vi "SYSKON P4500 Init Config.vi"() -> ()   [LabVIEW 2010]
panel:
  out "Output Current":string
  out "Output Voltage":string
  in  "Output State":bool=TRUE
  in  "Baud Rate":u32=19200
  in  "OCP Level":dbl=32.0 format="%.3f"
  in  "OVP Level":dbl=24.0 format="%.3f"
  in  "Instr. Descriptor":refnum<visa-resource-name>="COM4"
  out "error out":errorcluster {"code" format="%x"}
  in  "error in":errorcluster {"code" format="%x"}
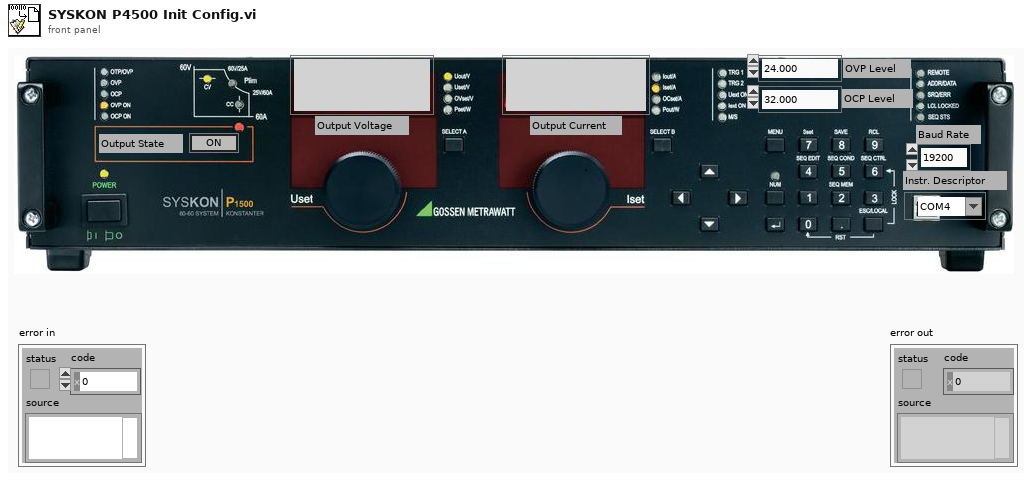
[diagram p1: front panel]
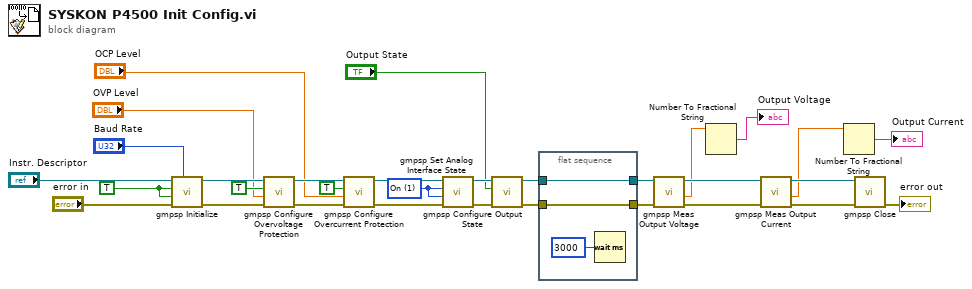
[diagram p0: block diagram]
diagram:
  w21 = 1 items=["Off", "On", "Signal State"] ("U ext (0: Off)")
  w31 = TRUE ("ID Query (True)")
  n1 = call <instrlib>:"gmpsp Initialize.vi"("Baud Rate"="Baud Rate", "error in"="error in", "Reset (True)"=w31, "ID Query (True)"=w31, "Instr. Descriptor"="Instr. Descriptor") -> ("error out"=w27:errorcluster, "VISA resource name out"=w29:refnum<visa-resource-name>)  [unwired: 5 in]
  n2 = call <instrlib>:"gmpsp Configure Overvoltage Protection.vi"("error in (no error)"=w27, "OVP Level (3.0 V)"="OVP Level", "OVP State (F: Off)"=TRUE, "VISA resource name"=w29) -> ("error out"=w24:errorcluster, "VISA resource name out"=w26:refnum<visa-resource-name>)  [unwired: 6 in]
  n3 = call <instrlib>:"gmpsp Configure Overcurrent Protection.vi"("error in (no error)"=w24, "OCP Level (22.0 A)"="OCP Level", "OCP State (F: Off)"=TRUE, "VISA resource name"=w26) -> ("error out"=w22:errorcluster, "VISA resource name out"=w23:refnum<visa-resource-name>)  [unwired: 6 in]
  n4 = call <instrlib>:"gmpsp Set Analog Interface State.vi"("error in (no error)"=w22, "I ext (0: Off)"=w21, "U ext (0: Off)"=w21, "VISA resource name"=w23) -> ("error out"=w18:errorcluster, "VISA resource name out"=w19:refnum<visa-resource-name>)  [unwired: 6 in]
  n5 = call <instrlib>:"gmpsp Configure Output State.vi"("error in (no error)"=w18, "Output State (F: Off)"="Output State", "VISA resource name"=w19) -> ("error out"=w11:errorcluster, "VISA resource name out"=w12:refnum<visa-resource-name>)  [unwired: 7 in]
  n6 = flat-sequence {
    tunnel: [w34] -> w13
    tunnel: w12 -> [w34]
    tunnel: w11 -> [w33]
    tunnel: [w33] -> w10
    frame #0 {
      n7 = Wait (ms)(milliseconds to wait=u32 3000) -> ()  [unwired: 1 out]
    }
  }
  n8 = call <instrlib>:"gmpsp Meas Output Voltage.vi"("error in (no error)"=w10, "VISA resource name"=w13) -> ("error out"=w16:errorcluster, "Output Voltage"=w9:dbl, "VISA resource name out"=w17:refnum<visa-resource-name>)  [unwired: 7 in]
  n9 = Number To Fractional String(number=w9) -> (F-format string=→"Output Voltage":string)  [unwired: 3 in]
  n10 = call <instrlib>:"gmpsp Meas Output Current.vi"("error in (no error)"=w16, "VISA resource name"=w17) -> ("error out"=w14:errorcluster, "Output Current"=w8:dbl, "VISA resource name out"=w15:refnum<visa-resource-name>)  [unwired: 7 in]
  n11 = Number To Fractional String(number=w8) -> (F-format string=→"Output Current":string)  [unwired: 3 in]
  n12 = call <instrlib>:"gmpsp Close.vi"("error in (no error)"=w14, "VISA resource name"=w15) -> ("error out"=→"error out":errorcluster)  [unwired: 9 in]
